vi "Enqueue At Front.vi"(6 "elements":T1[](array[typedef]), 8 "error in":errorcluster, 11 "queue in":refnum<queue>) -> (0 "error out":errorcluster, 3 "queue out":refnum<queue>)   [LabVIEW 2018]
doc: "This VI takes an array of elements and sequentially adds them to the front of a queue. Therefore, the last element in the array will be first in the queue."
uses:
  Exec Action.ctl
  Actions.ctl
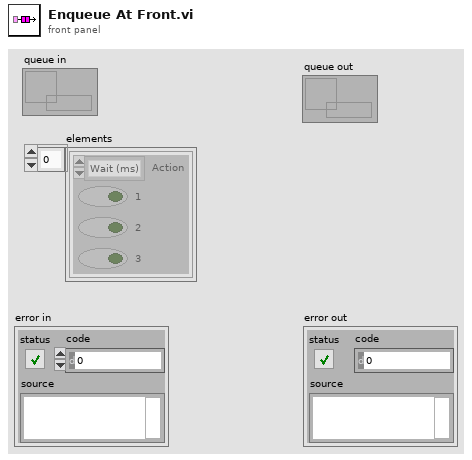
[diagram p1: front panel]
types:
  T1 = typedef "Exec Action.ctl" = cluster{"Action":T2, "1":bool, "2":bool, "3":bool}
  T2 = typedef "Actions.ctl" = enum16{"SW Init", "HW Init - Zaber", "HW Init - DO", "Init Asynch Vis", "Set Motion Params", "Set Zout Pos", "Set Zstart Pos", "Step Z", "Method close - Shear force", "Method close - SICM", "Method close - Keyence", "Method UI and HW init", "Tune Shear Force", "Plane Set Point 1", "Plane Set Point 2", "Plane Set Point 3", "Calculate Plane", "Scan UI", "Scan Ctrl", "Handle DLADS", "XY and Sensor Init", "Z Init", "MS Trig", "Line Motion", "Z Exit Ctrl", "MS Complete", "Pause Check Ctrl", "Shift Data", "Plot Profile", "Save Scan Config", "Save Profile Text File", "Wait (ms)", "Get Time", "HW Close - Zaber", "HW Close - DO", "Error", "Exit", "Shutdown Ctrl"}
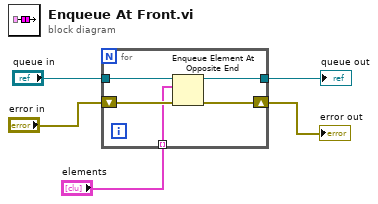
[diagram p0: block diagram]
diagram:
  n1 = for {
    tunnel: "queue in" -> [w10]
    tunnel: [w7] -> w4
    tunnel: "elements" -> [w6] mode=indexing
    shift-right: [w8] -> w1
    shift-left: "error in" -> [w9]
    n2 = Enqueue Element At Opposite End(queue=w10, element=w6, error in (no error)=w9) -> (queue out=w7:refnum<queue>, error out=w8:errorcluster)  [unwired: 1 in, 1 out]
  }
  "queue out" <- w4
  "error out" <- w1
